vi "Write Depth.vi"(8 "error in (no error)":errorcluster, 10 "Depth":dbl, 11 "Moving Ripple Noise in":refnum<class "Moving Ripple Noise.lvclass">) -> (0 "error out":errorcluster, 3 "Moving Ripple Noise out":refnum<class "Moving Ripple Noise.lvclass">)   [LabVIEW 2020, in "Moving Ripple Noise.lvclass"]
uses:
  Moving Ripple Noise.lvclass
  Moving Ripple Noise.lvclass/Moving Ripple Noise.ctl
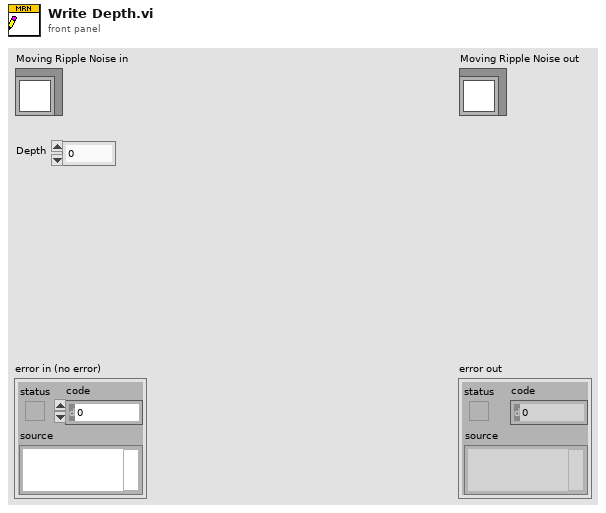
[diagram p1: front panel]
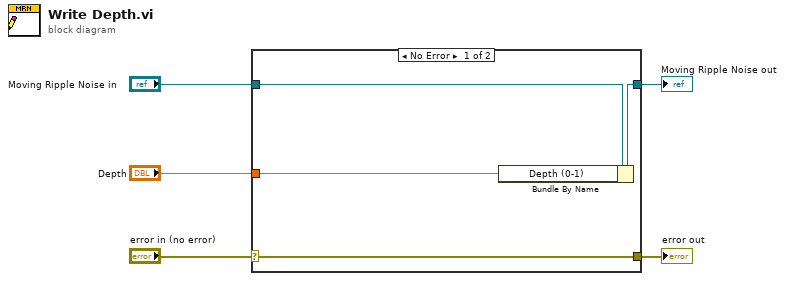
[diagram p0: block diagram]
diagram:
  n1 = case shown="No Error" "error in (no error)" {
    selector: "error in (no error)" -> [w9 w10]
    tunnel: [w9 w10] -> w4
    tunnel: [w7 w11] -> w2
    tunnel: "Moving Ripple Noise in" -> [w8 w11]
    tunnel: "Depth" -> [w6 _]
    frame No Error {
      n2 = Bundle By Name(cluster=w8, "Depth (0-1)"=w6) -> (w7:refnum<class "Moving Ripple Noise.lvclass">)
    }
    frame Error {
    }
  }
  "error out" <- w4
  "Moving Ripple Noise out" <- w2
